vi "Write DAQmx Task.vi"(8 "error in (no error)":errorcluster, 10 "DAQmx Task":refnum<k21>, 11 "PXI6521 in":refnum<class "PXI6521.lvclass">) -> (0 "error out":errorcluster, 3 "PXI6521 out":refnum<class "PXI6521.lvclass">)   [LabVIEW 2018, in "PXI6521.lvlib" / "PXI6521.lvclass"]
uses:
  PXI6521.lvclass
  PXI6521.lvclass/PXI6521.ctl
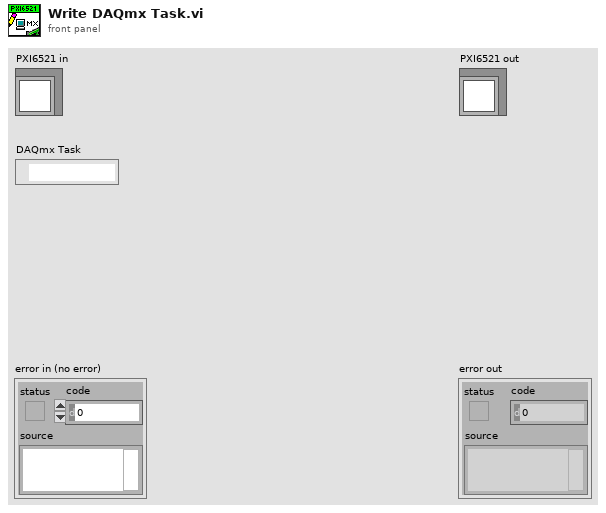
[diagram p1: front panel]
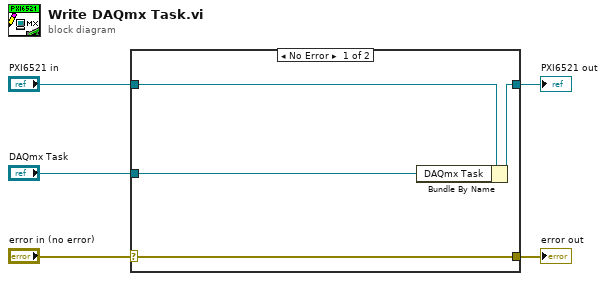
[diagram p0: block diagram]
diagram:
  n1 = case shown="No Error" "error in (no error)" {
    selector: "error in (no error)" -> [w9 w10]
    tunnel: [w9 w10] -> w4
    tunnel: [w7 w11] -> w2
    tunnel: "PXI6521 in" -> [w8 w11]
    tunnel: "DAQmx Task" -> [w6 _]
    frame No Error {
      n2 = Bundle By Name(cluster=w8, "DAQmx Task"=w6) -> (w7:refnum<class "PXI6521.lvclass">)
    }
    frame Error {
    }
  }
  "error out" <- w4
  "PXI6521 out" <- w2
